vi "OFBS_train_ANN.vi"(6 "Train Data":T1, 8 "error in (no error)":errorcluster, 9 "# of hidden neurons":i32=2, 10 "Parameters":i32[](array[numeric]), 11 "OFBS class in":refnum<class "OptFreqBandsSearch.lvclass">) -> (0 "error out":errorcluster, 1 "exit flag":i32, 2 "ANN out":T2={"Training Data"={"dim in"=0, "dim out"=0, "# samples"=0, "Input"=[], "Output"=[]}, "Normalize Info"={"input min"=[], "input max"=[], "output min"=[], "output max"=[]}, "3-layer NN"={"# input neuron "=0, "# hidden neuron"=0, "# output neuron"=0, "Weight (I->H)"=[], "Weight (H->O)"=[], "Output"=[], "Hidden Out"=[], "Derivation Output"=[], "Derivation Hidden"=[], "dw (I->H)"=[], "dw (H->O)"=[]}, "Ternimal Condition"={"min MSE"=1e-05, "min delta MSE"=1e-05, "min step length"=1e-08, "max iteration"=inf}}, 3 "OFBS class out":refnum<class "OptFreqBandsSearch.lvclass">)   [LabVIEW 2016, in "Optimal Frequency Bands Search.lvlib" / "OptFreqBandsSearch.lvclass"]
doc: "Метод, реализующий построение классификатора на основе многослойного персептрона. Для обучения классификатора используются обучающие данные."
uses:
  OptFreqBandsSearch.lvclass
  <vilib>/addons/Machine Learning/Supervised Learning/ml_BP_Project.ctl
  <vilib>/addons/Machine Learning/Supervised Learning/ml_BP_Data.ctl
  <vilib>/addons/Machine Learning/Supervised Learning/ml_BP_Normalize Data.ctl
  <vilib>/addons/Machine Learning/Supervised Learning/ml_BP_3layer Feedforward.ctl
  <vilib>/addons/Machine Learning/Supervised Learning/ml_BP_Terminal Condition.ctl
  OFBS_DataTypes.ctl
  OptFreqBandsSearch.lvclass/OptFreqBandsSearch.ctl
  Optimal Frequency Bands Search.lvlib
  <vilib>/addons/Machine Learning/NILabs_MLT.lvlib
panel:
  # "This VI is a part of BCI Design library, http://www.ru-bci.org \nCopyright © 2020, Sotnikov Peter, All rights reserved. License: CC BY-NC 4.0"
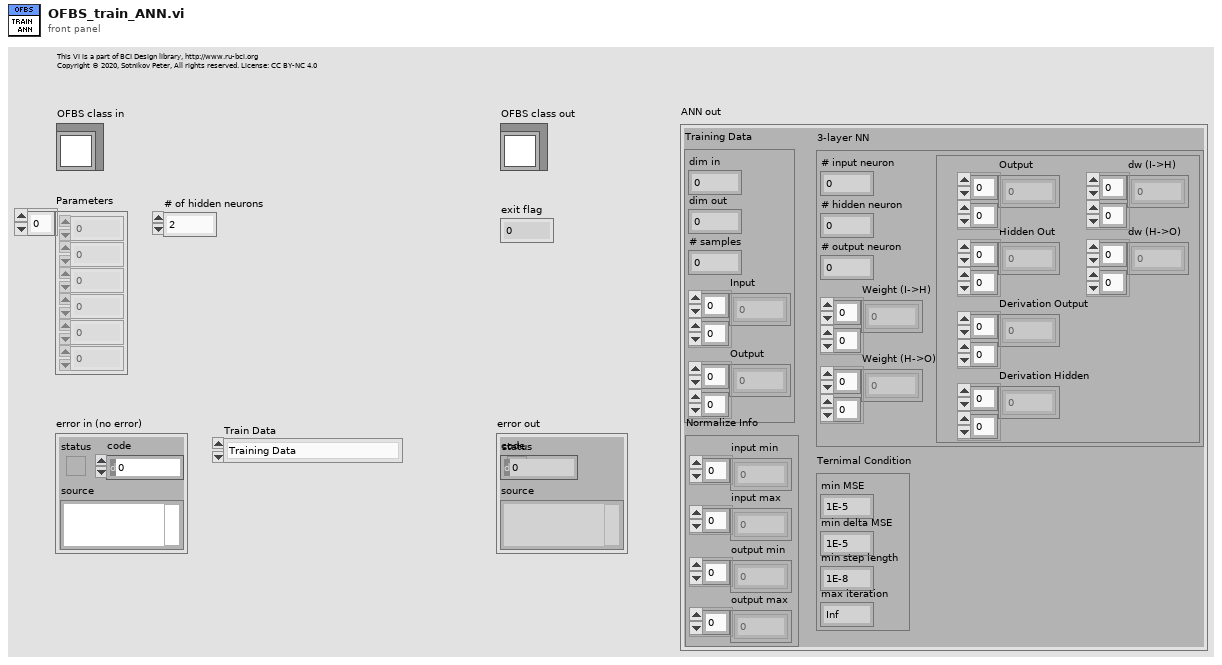
[diagram p1: front panel]
types:
  T1 = typedef "Optimal Frequency Bands Search.lvlib/OFBS_DataTypes.ctl" = enum16{"Training Data", "Test Data", "Training Data (cross-check)", "Test Data (cross-check)"}
  T2 = typedef "NILabs_MLT.lvlib/ml_BP_Project.ctl" = cluster{"Training Data":T3, "Normalize Info":T4, "3-layer NN":T5, "Ternimal Condition":T6}
  T3 = typedef "NILabs_MLT.lvlib/ml_BP_Data.ctl" = cluster{"dim in":i32, "dim out":i32, "# samples":i32, "Input":dbl[][], "Output":dbl[][]}
  T4 = typedef "NILabs_MLT.lvlib/ml_BP_Normalize Data.ctl" = cluster{"input min":dbl[], "input max":dbl[], "output min":dbl[], "output max":dbl[]}
  T5 = typedef "NILabs_MLT.lvlib/ml_BP_3layer Feedforward.ctl" = cluster{"# input neuron ":i32, "# hidden neuron":i32, "# output neuron":i32, "Weight (I->H)":dbl[][], "Weight (H->O)":dbl[][], "Output":dbl[][], "Hidden Out":dbl[][], "Derivation Output":dbl[][], "Derivation Hidden":dbl[][], "dw (I->H)":dbl[][], "dw (H->O)":dbl[][]}
  T6 = typedef "NILabs_MLT.lvlib/ml_BP_Terminal Condition.ctl" = cluster{"min MSE":dbl, "min delta MSE":dbl, "min step length":dbl, "max iteration":dbl}
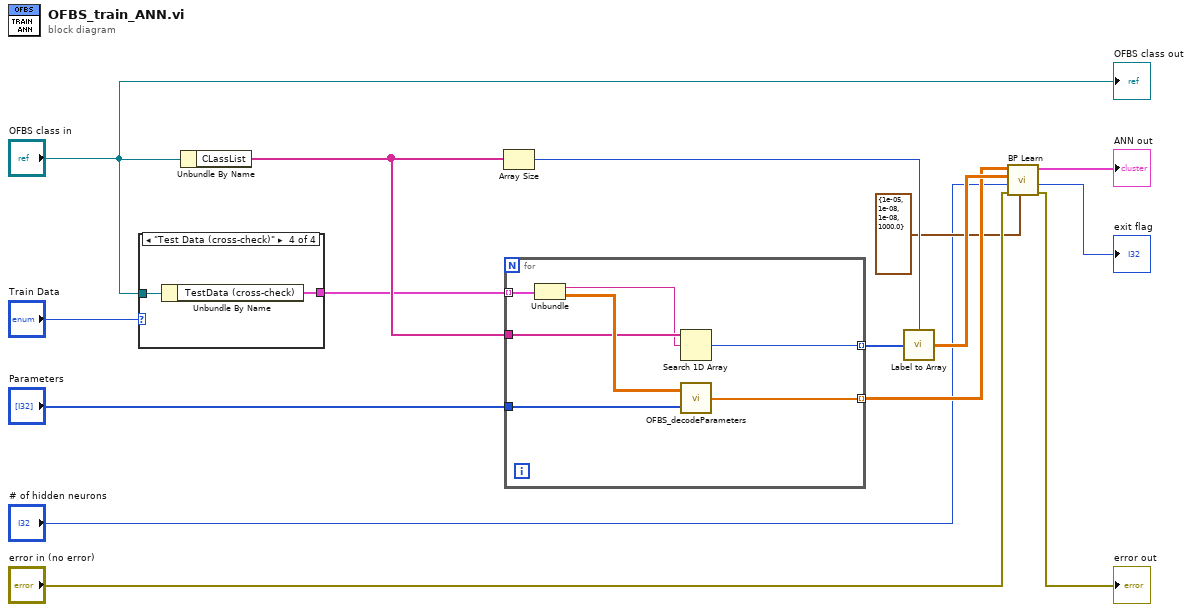
[diagram p0: block diagram]
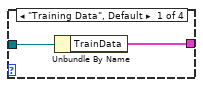
[diagram p2: hidden frame]
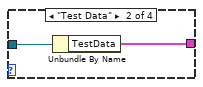
[diagram p3: hidden frame]
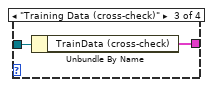
[diagram p4: hidden frame]
diagram:
  n1 = case shown="\"Test Data (cross-check)\"" "Train Data" {
    tunnel: "OFBS class in" -> [w17 w19 w21 w23]
    tunnel: [w16 w18 w20 w22] -> w2
    frame "Training Data", Default {
      n2 = Unbundle By Name(w17) -> ("TrainData"=w16:cluster{"ClassLabel":string, "Trial":dbl[][]}[])
    }
    frame "Test Data" {
      n3 = Unbundle By Name(w19) -> ("TestData"=w18:cluster{"ClassLabel":string, "Trial":dbl[][]}[])
    }
    frame "Training Data (cross-check)" {
      n4 = Unbundle By Name(w21) -> ("TrainData (cross-check)"=w20:cluster{"ClassLabel":string, "Trial":dbl[][]}[])
    }
    frame "Test Data (cross-check)" {
      n5 = Unbundle By Name(w23) -> ("TestData (cross-check)"=w22:cluster{"ClassLabel":string, "Trial":dbl[][]}[])
    }
  }
  n6 = Unbundle By Name("OFBS class in") -> ("CLassList"=w14:string[])
  n7 = Array Size(array=w14) -> (size(s)=w10:i32)
  n8 = for {
    tunnel: w2 -> [w30] mode=indexing
    tunnel: "Parameters" -> [w28]
    tunnel: w14 -> [w27]
    tunnel: [w24] -> w8 mode=indexing
    tunnel: [w25] -> w11 mode=indexing
    n9 = Unbundle(w30) -> ("ClassLabel"=w26:string, "Trial"=w29:dbl[][])
    n10 = Search 1D Array(1D array=w27, element=w26) -> (index of element=w25:i32)  [unwired: 1 in]
    n11 = call "OFBS_decodeParameters.vi"("Parameters"=w28, "Trial"=w29) -> ("FeatureVector"=w24:dbl[])
  }
  n12 = call <vilib>:"Label to Array.vi"("Classes"=w11, "# of classes"=w10) -> ("Array"=w9:dbl[][])
  n13 = call <vilib>:"BP Learn.vi"("Stopping Criteria"=T6 {"min MSE"=1e-05, "min delta MSE"=1e-08, "min step length"=1e-08, "max iteration"=1000.0}, "error in (no error)"="error in (no error)", "# of hidden neuron"="# of hidden neurons", "Training outputs"=w9, "Training data samples"=w8) -> ("error out"=→"error out":errorcluster, "exit flag"=→"exit flag":i32, "BP Project"=→"ANN out":T2)  [unwired: 3 in, 1 out]
  "OFBS class out" <- "OFBS class in"
